vi "FTW-Test.vi"() -> ()   [LabVIEW 2014]
uses:
  src/core/time/FTW-Time-DisplayFormat-Timestamp.ctl
  src/core/error/FTW-ERR-ExceptionType.ctl
  src/core/time/FTW-Time-Uptime.vi
  src/core/reflection/FTW-Reflection-Type.vi
  lib/jansson/FTWLib-JSON-LibraryFilepath.vi
  src/core/json/lib/FTW-JSON-Core-LibraryError.vi
  src/core/json/lib/FTW-JSON-Core-ElementType.vi
  src/core/error/FTW-ERR-ThrowGenericError.vi
  src/core/json/lib/FTW-JSON-Core-EncodingFlags.vi
  src/core/error/FTW-ERR-ThrowError.vi
  src/core/error/FTW-ERR-CallChain.vi
  src/core/string/FTW-STR-ReplaceWhitespace.vi
  src/core/json/lib/FTW-JSON-Core-GetFlattenedValue.vi
  src/core/sync/barrier/FTW-Sync-Synchronizer.xnode
  src/core/json/FTW-JSON-Deserialize/FTW-JSON-Deserialize.xnode
  src/core/array/shuffle/FTW-Array-Shuffle.xnode
  <vilib>/regexp/Match Regular Expression.xnode
  kernel32.dll
panel:
  out "Results":string
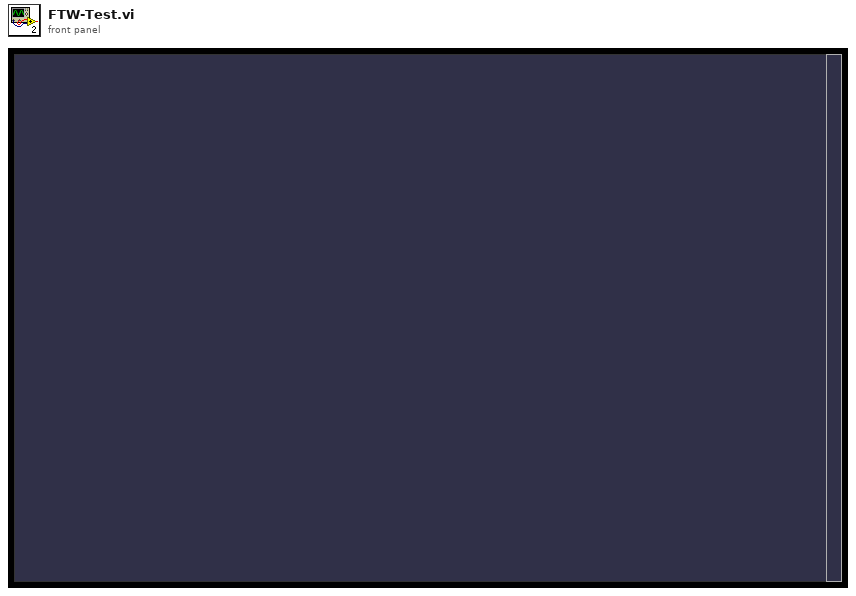
[diagram p1: front panel]
types:
  T1 = typedef "FTW-Time-DisplayFormat-Timestamp.ctl" = enum16{"YYYY-MM-DDT00:00:00.000Z (ISO-8601)", "YYYY-MM-DDT00-00-00Z (Simple ISO-8601)", "YYYY-MM-DD"}
  T2 = cluster{"Randomize Test Order":bool, "Tests Directory":path, "Test Configuration":cluster{"Default":cluster{"Enable":bool, "Iterations":i32}}, "Test Configuration":string, "Test Worker Pool Size":i32}
  T3 = enum32{"invalid app kind", "Development System", "Run Time System", "Student Edition", "Embedded LabVIEW", "Evaluation", "Custom"}
  T4 = enum32{"invalid CPU target", "Motorola 68K", "PowerPC", "Intel x86", "SPARC", "PA-RISC", "MIPS", "Alpha", "ARM", "AMD/Intel x64"}
  T5 = typedef "FTW-ERR-ExceptionType.ctl" = enum16{"OK", "Info", "Warning", "Error"}
  T6 = cluster{"Execute?":bool, "TestName":string, "MinTime":dbl, "MeanTime":dbl, "MaxTime":dbl, "Runs":i32, "Result":T5, "Hint":string, "TotalTime":dbl}
  T7 = enum32{"Bad", "Idle", "Run top level", "Running"}
  T8 = cluster{"VIRef":refnum<vi>, "TestName":string, "TestInstance":i32, "TestPoolSize":i32, "TestID":i32}
  T9 = cluster{"Color":u32, "Text":string, "Comment":string}[]
  T10 = cluster{"Color":u32, "Text":string, "Comment":string}
  T11 = cluster{u32, "offset past match":u32, "Color":u32}[]
  T12 = cluster{"VIRef":refnum<vi>, "TestName":string, "TestInstance":i32, "TestPoolSize":i32, "TestID":i32}[]
  T13 = cluster{"TestID":i32, "ElapsedTime":dbl, "Result":T5}
  T14 = cluster{"Execute?":bool, "TestName":string, "MinTime":dbl, "MeanTime":dbl, "MaxTime":dbl, "Runs":i32, "Result":T5, "Hint":string, "TotalTime":dbl}[]
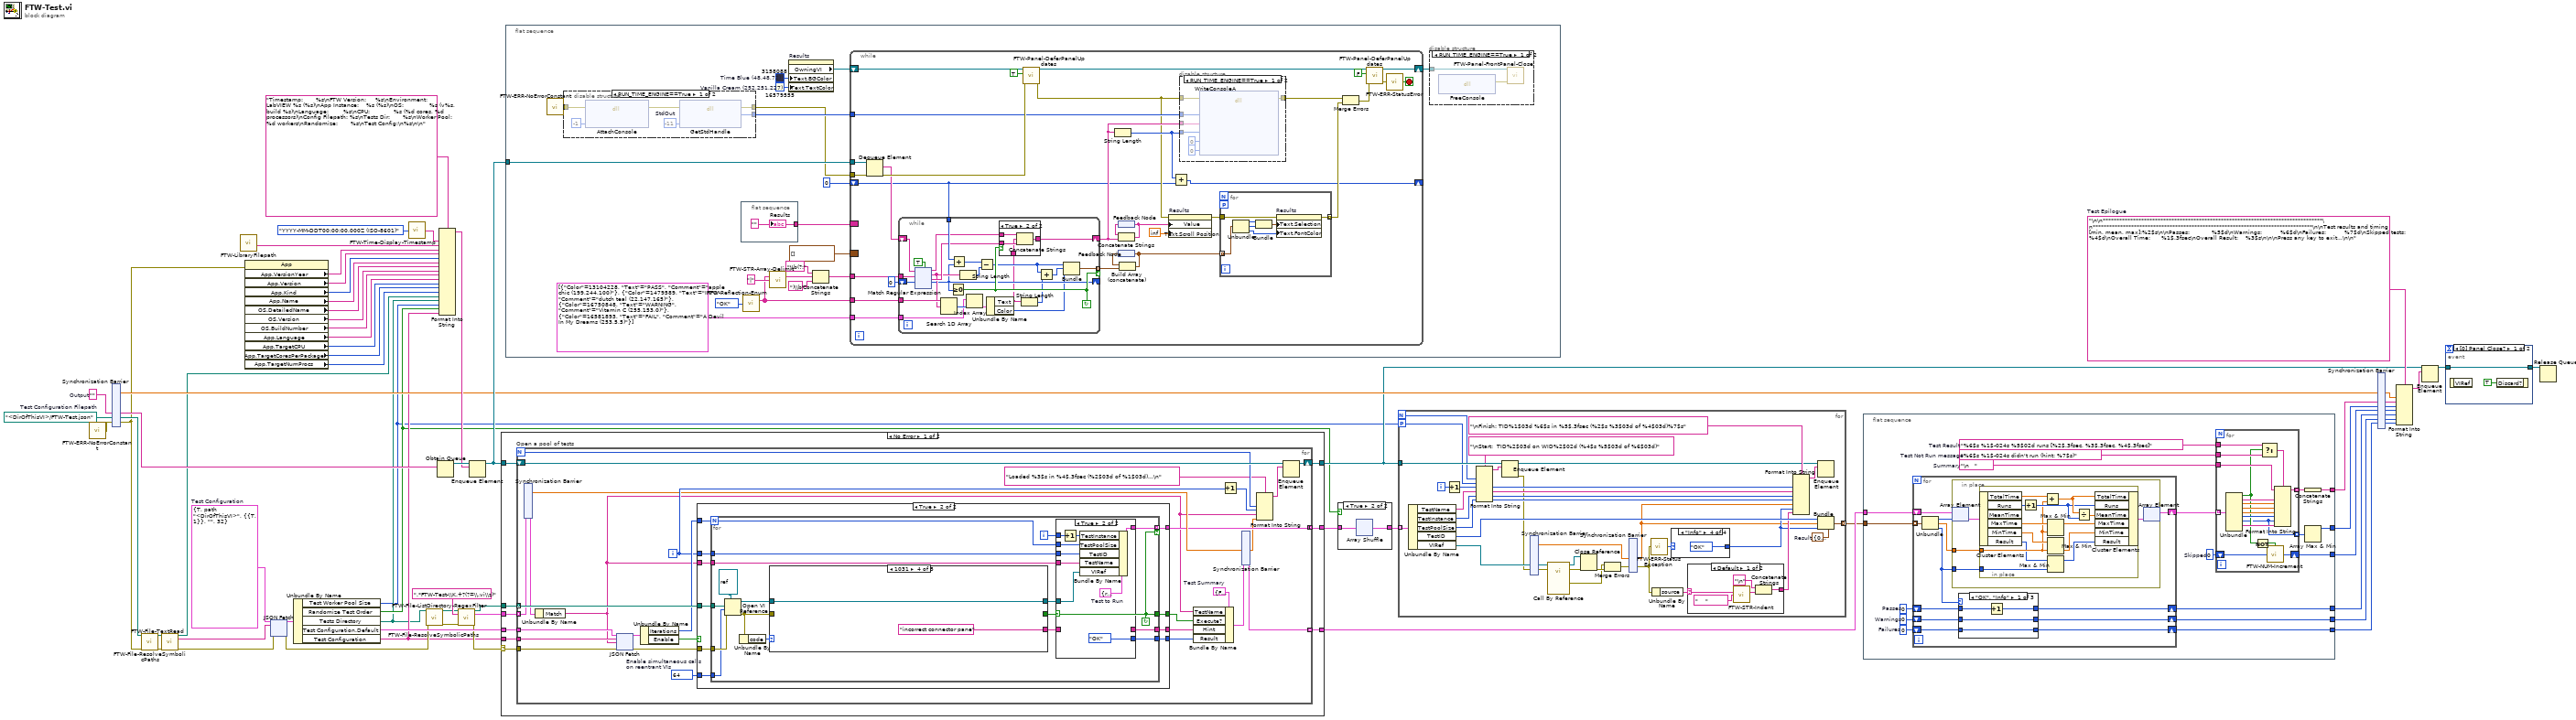
[diagram p0: block diagram]
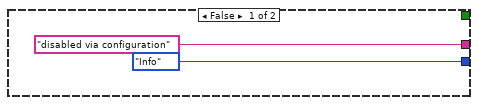
[diagram p5: hidden frame]
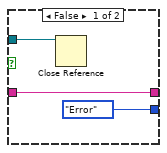
[diagram p6: hidden frame]
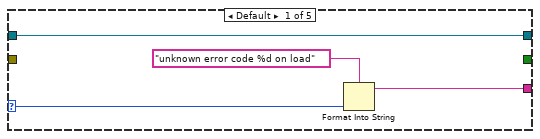
[diagram p7: hidden frame]
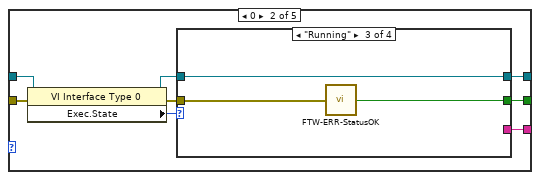
[diagram p8: hidden frame]
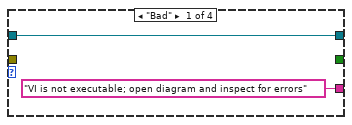
[diagram p9: hidden frame]
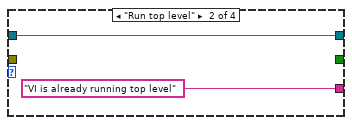
[diagram p10: hidden frame]
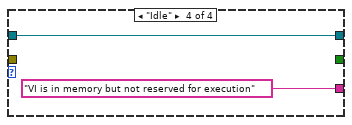
[diagram p11: hidden frame]
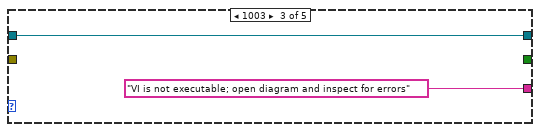
[diagram p12: hidden frame]
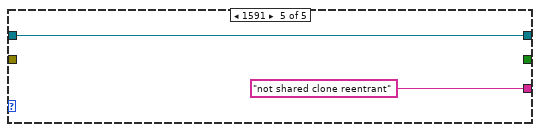
[diagram p13: hidden frame]
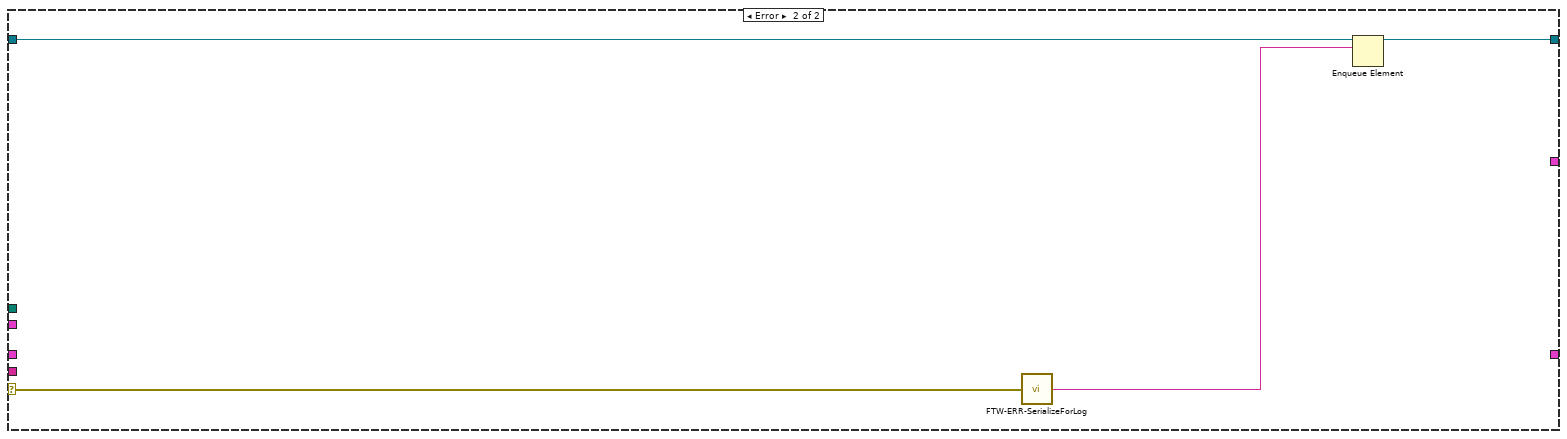
[diagram p14: hidden frame]
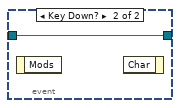
[diagram p19: hidden frame]
diagram:
  w55 = "\n\n********************************************************************************\n********************************************************************************\n\nTest results and timing [min, mean, max]:%2$s\n\nPasses:            %5$d\nWarnings:          %6$d\nFailures:          %7$d\nSkipped tests:     %4$d\nOverall Time:      %1$.3fsec\nOverall Result:    %3$s\n\n\nPress any key to exit...\n\n"  # Test Epilogue
  w38 = path "<DirOfThisVI>/FTW-Test.json"  # Test Configuration Filepath
  w35 = T2 {"Randomize Test Order"=TRUE, "Tests Directory"=path "<DirOfThisVI>", "Test Configuration"={"Default"={"Enable"=TRUE, "Iterations"=1}}, "Test Configuration"="", "Test Worker Pool Size"=32}  # Test Configuration
  w39 = ""  # Output
  n1 = call "FTW-ERR-NoErrorConstant.vi"() -> ("no error"=w11:errorcluster)
  n2 = xnode "Synchronization Barrier"("Synchronized Signal 1"=w39, "Synchronized Signal 2"=w38, "Synchronized Signal 3"=w11) -> ("High-Resolution Timer"=w16:dbl, w36:string, w37:path, w10:errorcluster)  [unwired: 1 in, 1 out]
  n3 = call "FTW-File-ResolveSymbolicPaths.vi"("Unresolved Path"=w37, "error in"=w10) -> ("Resolved Path"=w18:path, "error out"=w56:errorcluster)  [unwired: 12 in]
  n4 = call "FTW-File-TextRead.vi"("Filepath"=w18, "error in"=w56) -> ("Filepath out"=w8:path, "Text"=w31:string, "error out"=w33:errorcluster)  [unwired: 11 in]
  n5 = call "FTW-LibraryFilepath.vi"() -> ("Library Version"=w6:string)  [unwired: 9 in, 2 out]
  n6 = property class="App"(error in=w10) -> ("App.VersionYear"=w30:string, "App.Version"=w28:string, "App.Kind"=w20:T3, "App.Name"=w19:string, "OS.DetailedName"=w29:string, "OS.Version"=w27:string, "OS.BuildNumber"=w26:string, "App.Language"=w25:string, "App.TargetCPU"=w24:T4, "App.TargetCoresPerPackage"=w23:i32, "App.TargetNumProcs"=w21:i32)  [unwired: 1 in, 2 out]
  n7 = xnode "JSON Fetch"("Type and Defaults"=w35, "JSON String"=w31, "error in"=w33) -> ("Values"=w34:T2, "error out"=w32:errorcluster)  [unwired: 1 in]
  n8 = Unbundle By Name(w34) -> ("Test Worker Pool Size"=w3:i32, "Randomize Test Order"=w7:bool, "Tests Directory"=w4:path, "Test Configuration.Default"=w61:cluster{"Enable":bool, "Iterations":i32}, "Test Configuration"=w9:string)
  n9 = call "FTW-Time-Display-Timestamp.vi"("Format"=FTW-Time-DisplayFormat-Timestamp."YYYY-MM-DDT00:00:00.000Z (ISO-8601)") -> ("Formatted Timestamp"=w15:string)  [unwired: 3 in]
  n10 = call "FTW-File-ResolveSymbolicPaths.vi"("Unresolved Path"=w4, "error in"=w32) -> ("Resolved Path"=w5:path, "error out"=w62:errorcluster)  [unwired: 12 in]
  n11 = Obtain Queue(element data type=w36) -> (queue out=w57:refnum<queue>)  [unwired: 4 in, 2 out]
  n12 = Format Into String(format string="Timestamp:       %s\nFTW Version:     %s\nEnvironment:     LabVIEW %s (%s)\nApp Instance:    %s (%s)\nOS:              %s (v%s, build %s)\nLanguage:        %s\nCPU:             %s (%d cores, %d processors)\nConfig Filepath: %s\nTests Dir:       %s\nWorker Pool:     %d workers\nRandomize:       %s\nTest Config:\n%s\n\n", w15, w6, w30, w28, w20, w19, w29, w27, w26, w25, w24, w23, w21, w8, w4, w3, w7, w9) -> (resulting string=w17:string)  [unwired: 2 in, 1 out]
  n13 = call "FTW-File-ListDirectory-RegexFilter.vi"("Directory to Search"=w5, "Filename Regex Filter"=".*FTW-Test-\\K.+?(?=\\.vi\\z)", "error in"=w62) -> ("Matching Filepaths"=w64:path[], "Regex Results"=w65:cluster{"Match":string, "Submatches":string[]}[], "error out"=w54:errorcluster)  [unwired: 9 in, 1 out]
  n14 = Enqueue Element(queue=w57, element=w17) -> (queue out=w53:refnum<queue>)  [unwired: 2 in, 2 out]
  n15 = case shown="No Error" w54 {
    selector: w54 -> [w71 w253]
    tunnel: w65 -> [w75 _]
    tunnel: w64 -> [w74 _]
    tunnel: [w67 _] -> w12
    tunnel: w61 -> [w73 _]
    tunnel: w9 -> [w72 _]
    tunnel: [w70 _] -> w60
    tunnel: w53 -> [w69 w250]
    tunnel: [w68 w252] -> w13
    frame No Error {
      n16 = for "Open a pool of tests" {
        N -> [w97]
        tunnel: w71 -> [w93]
        tunnel: [w87] -> w67 mode=concatenating
        tunnel: w75 -> [w90] mode=indexing
        tunnel: w74 -> [w103] mode=indexing
        tunnel: [w85] -> w70 mode=indexing
        tunnel: w73 -> [w95]
        tunnel: w72 -> [w94]
        shift-right: [w83] -> w68
        shift-left: w69 -> [w99]
        i -> [w96]
        w81 = 64  # Enable simultaneous calls on reentrant VIs
        w100 = T6 {"Execute?"=FALSE, "TestName"="", "MinTime"=inf, "MeanTime"=0.0, "MaxTime"=-inf, "Runs"=0, "Result"=enum."OK", "Hint"="", "TotalTime"=0.0}  # Test Summary
        n17 = xnode "Synchronization Barrier"("Synchronized Signal 1"=w90) -> ("High-Resolution Timer"=w88:dbl, w89:cluster{"Match":string, "Submatches":string[]})  [unwired: 1 in, 1 out]
        n18 = Unbundle By Name(w89) -> ("Match"=w78:string)
        n19 = xnode "JSON Fetch"("Type and Defaults"=w95, "JSON String"=w94, "Element Path"=w78, "error in"=w93) -> ("Values"=w91:cluster{"Enable":bool, "Iterations":i32}, "error out"=w92:errorcluster)
        n20 = Unbundle By Name(w91) -> ("Iterations"=w101:i32, "Enable"=w77:bool)
        n21 = case shown="True" w77 {
          tunnel: w103 -> [_ w193]
          tunnel: w81 -> [_ w192]
          tunnel: [_ w191] -> w87
          tunnel: w96 -> [_ w190]
          tunnel: ["disabled via configuration" w189] -> w102
          tunnel: w101 -> [_ w188]
          tunnel: w92 -> [_ w187]
          tunnel: w78 -> [_ w186]
          tunnel: [FTW-ERR-ExceptionType."Info" ("Result") w185] -> w82
          tunnel: [_ w184] -> w76
          frame False {
          }
          frame True {
            n22 = for {
              N: w188 -> [w202]
              tunnel: w187 -> [w210]
              tunnel: w193 -> [w209]
              tunnel: w192 -> [w208]
              tunnel: w186 -> [w204]
              tunnel: [w201] -> w191 mode=indexing if=w194
              tunnel: [w197] -> w189
              tunnel: w190 -> [w196]
              tunnel: [w195] -> w185
              tunnel: [w194] -> w184
              i -> [w203]
              stop <- w194 continue-if-true
              n23 = Open VI Reference(type specifier VI Refnum (for type only)=refnum<vi> refnum, vi path=w209, options=w208, error in (no error)=w210) -> (vi reference=w200:refnum<vi>, error out=w206:errorcluster)  [unwired: 2 in]
              n24 = Unbundle By Name(w206) -> ("code"=w205:i32)
              n25 = case shown="1031" w205 {
                selector: w205 -> [w225 _ _ _ _]
                tunnel: w200 -> [w223 w234 w244 w246 w248]
                tunnel: w206 -> [_ w233 _ _ _]
                tunnel: [_ w230 _ _ _] -> w194
                tunnel: [w224 w228 "VI is not executable; open diagram and inspect for errors" "incorrect connector pane" "not shared clone reentrant"] -> w198
                tunnel: [w223 w227 w244 w246 w248] -> w199
                frame Default {
                  n26 = Format Into String(format string="unknown error code %d on load", w225) -> (resulting string=w224:string)  [unwired: 2 in, 1 out]
                }
                frame 0 {
                  n27 = property class="VI Interface Type 0"(reference=w234, error in=w233) -> (reference out=w231:refnum<vi>, error out=w232:errorcluster, "Exec.State"=w229:T7)
                  n28 = case shown="\"Running\"" w229 {
                    tunnel: w232 -> [_ _ w240 _]
                    tunnel: w231 -> [w235 w237 w241 w243]
                    tunnel: [_ _ w239 _] -> w230
                    tunnel: ["VI is not executable; open diagram and inspect for errors" "VI is already running top level" _ "VI is in memory but not reserved for execution"] -> w228
                    tunnel: [w235 w237 w241 w243] -> w227
                    frame "Bad" {
                    }
                    frame "Run top level" {
                    }
                    frame "Running" {
                      n29 = call "FTW-ERR-StatusOK.vi"("error to check"=w240) -> ("Status OK?"=w239:bool)
                    }
                    frame "Idle" {
                    }
                  }
                }
                frame 1003 {
                }
                frame 1031 {
                }
                frame 1591 {
                }
              }
              n30 = case shown="True" w194 {
                tunnel: w199 -> [w213 w222]
                tunnel: w204 -> [_ w216]
                tunnel: w203 -> [_ w221]
                tunnel: w202 -> [_ w219]
                tunnel: [_ w220] -> w201
                tunnel: w198 -> [w212 _]
                tunnel: [w212 _] -> w197
                tunnel: w196 -> [_ w218]
                tunnel: [FTW-ERR-ExceptionType."Error" ("Result") FTW-ERR-ExceptionType."OK" ("Result")] -> w195
                frame False {
                  n31 = Close Reference(reference=w213) -> ()  [unwired: 1 in, 1 out]
                }
                frame True {
                  w217 = T8 {"VIRef"=refnum, "TestName"="", "TestInstance"=0, "TestPoolSize"=0, "TestID"=0}  # Test to Run
                  n32 = Increment(x=w221) -> (x+1=w215:i32)
                  n33 = Bundle By Name(cluster=w217, "TestInstance"=w215, "TestPoolSize"=w219, "TestID"=w218, "TestName"=w216, "VIRef"=w222) -> (w220:T8)
                }
              }
            }
          }
        }
        n34 = Bundle By Name(cluster=w100, "TestName"=w78, "Execute?"=w76, "Hint"=w102, "Result"=w82) -> (w86:T6)
        n35 = Increment(x=w96) -> (x+1=w79:i32)
        n36 = xnode "Synchronization Barrier"("Upstream Timer Value"=w88, "Synchronized Signal 1"=w86) -> ("Elapsed Time"=w84:dbl, w85:T6)  [unwired: 1 out]
        n37 = Format Into String(format string="Loaded %3$s in %4$.3fsec (%2$03d of %1$03d)...\n", w97, w79, w78, w84) -> (resulting string=w98:string)  [unwired: 2 in, 1 out]
        n38 = Enqueue Element(queue=w99, element=w98) -> (queue out=w83:refnum<queue>)  [unwired: 2 in, 2 out]
      }
    }
    frame Error {
      n39 = call "FTW-ERR-SerializeForLog.vi"("error in"=w253) -> ("Serialized Error"=w251:string)
      n40 = Enqueue Element(queue=w250, element=w251) -> (queue out=w252:refnum<queue>)  [unwired: 2 in, 2 out]
    }
  }
  n41 = flat-sequence {
    tunnel: w53 -> [w272]
    frame #0 {
      w268 = u32 16579555  # Vanilla Cream (252,251,227)
      w269 = u32 3158088  # Time Blue (48,48,72)
      n42 = call "FTW-ERR-NoErrorConstant.vi"() -> ("no error"=w257:errorcluster)
      n43 = disable-structure shown="RUN_TIME_ENGINE==True" {
        disable-tunnel: w257 -> [w278 w282]
        disable-tunnel: [w277 w282] -> w254
        disable-tunnel: [w276 _] -> w260
        frame condition #0 {
          w280 = -11  # StdOut
          n44 = dll-call lib="kernel32.dll" fn="AttachConsole"(error in=w278, "arg1"=-1) -> (error out=w281:errorcluster)  [unwired: 4 in, 1 out]
          n45 = dll-call lib="kernel32.dll" fn="GetStdHandle"(error in=w281, "nStdHandle"=w280) -> (error out=w277:errorcluster, "return type"=w276:i32)  [unwired: 3 in, 1 out]
        }
        frame condition #1 (active) {
        }
      }
      n46 = flat-sequence {
        tunnel: [w275] -> w258
        frame #0 {
          w275 = "" ("Results")
          "Results" <- w275
        }
      }
      n47 = call "FTW-Reflection-Enum.vi"("Enum"=FTW-ERR-ExceptionType."OK" ("Exception")) -> ("Enum Items"=w262:string[])  [unwired: 12 in, 2 out]
      n48 = call "FTW-STR-Array-Delimit.vi"("Array of Strings"=w262, "Delimiter"="|") -> ("Delimited String"=w264:string)  [unwired: 13 in]
      n49 = property on="Results" class="Str"("Text.BGColor"=w269, "Text.TextColor"=w268) -> ("OwningVI"=w267:refnum<vi>)  [unwired: 2 in, 2 out]
      n50 = Concatenate Strings("\\b(?:" ("string"), w264, ")\\b" ("string")) -> (w263:string)
      n51 = while {
        tunnel: w260 -> [w300]
        tunnel: w263 -> [w311]
        border: cluster{u32, "offset past match":u32, u32}[] [] -> [_]
        border: w258 -> [_]
        tunnel: w262 -> [w310]
        tunnel: T9 [{"Color"=13104228, "Text"="PASS", "Comment"="apple chic (199,244,100)"}, {"Color"=1479589, "Text"="INFO", "Comment"="dutch teal (22,147,165)"}, {"Color"=16750848, "Text"="WARNING", "Comment"="Vitamin C (255,153,0)"}, {"Color"=16581893, "Text"="FAIL", "Comment"="A Devil In My Dreams (253,5,5)"}] -> [w298]
        shift-right: [w297] -> w259
        shift-left: w267 -> [w309]
        tunnel: w272 -> [w313]
        tunnel: w254 -> [w293]
        shift-right: [w284] -> _
        shift-left: 0 ("length") -> [w285]
        stop <- w296 stop-if-true
        n52 = Dequeue Element(queue=w313, error in (no error)=w293) -> (element=w295:string, error out=w312:errorcluster)  [unwired: 1 in, 2 out]
        n53 = while {
          shift-right: [w336] -> _
          shift-left: 0 ("offset past match") -> [w350]
          tunnel: w311 -> [w351]
          tunnel: [w345] -> w306 mode=indexing if=w340
          tunnel: w285 -> [w348]
          tunnel: w310 -> [w347]
          shift-right: [w342] -> w299
          shift-left: w295 -> [w344]
          tunnel: w298 -> [w338]
          stop <- w340 continue-if-true
          n54 = xnode "Match Regular Expression"("input string"=w344, "regular expression"=w351, "offset (0)"=w350, "multiline? (F)"=TRUE) -> ("before match"=w343:string, "whole match"=w337:string, "after match"=w341:string, "offset past match"=w336:i32)  [unwired: 2 in, 1 out]
          n55 = Search 1D Array(1D array=w347, element=w337) -> (index of element=w339:i32)  [unwired: 1 in]
          n56 = Greater Or Equal To 0?(x=w336) -> (x >= 0?=w340:bool)
          n57 = Add(x=w348, y=w336) -> (x+y=w346:i32)
          n58 = String Length(string=w337) -> (length=w335:i32)
          n59 = Index Array(array=w338, index=w339) -> (element=w331:T10)
          n60 = Subtract(x=w346, y=w335) -> (x-y=w334:i32)
          n61 = Unbundle By Name(w331) -> ("Text"=w330:string, "Color"=w329:u32)
          n62 = case shown="True" w340 {
            tunnel: w343 -> [w352 w356]
            tunnel: [w352 w355] -> w342
            tunnel: w341 -> [_ w354]
            tunnel: w330 -> [_ w353]
            frame False {
            }
            frame True {
              n63 = Concatenate Strings(w356, w353, w354) -> (w355:string)
            }
          }
          n64 = String Length(string=w330) -> (length=w332:i32)
          n65 = Add(x=w334, y=w332) -> (x+y=w333:i32)
          n66 = Bundle(w334, w333, "Color"=w329) -> (w345:cluster{i32, i32, "Color":u32})  [unwired: 1 in]
        }
        n67 = call "FTW-Panel-DeferPanelUpdates.vi"("error in"=w312, "Defer?"=TRUE, "VI Ref"=w309) -> ("error out"=w290:errorcluster, "VI Ref out"=w302:refnum<vi>)  [unwired: 7 in]
        n68 = String Length(string=w299) -> (length=w292:i32)
        n69 = feedback #1() -> (w304:string)
        n70 = Concatenate Strings(w304, w299) -> (w305:string)
        n71 = feedback-in #1(w305) -> ()
        n72 = feedback #2() -> (w307:cluster{u32, "offset past match":u32, u32}[])
        n73 = Build Array (concatenate)(w307, w306) -> (w291:T11)
        n74 = feedback-in #2(w291) -> ()
        n75 = property on="Results" class="Str"(error in=w290, "Value"=w305, "Text.Scroll Position"=inf) -> (error out=w289:errorcluster)  [unwired: 1 in, 1 out]
        n76 = Add(x=w292, y=w285) -> (x+y=w284:i32)
        n77 = disable-structure shown="RUN_TIME_ENGINE==True" {
          disable-tunnel: w300 -> [w318 _]
          disable-tunnel: [w317 w321] -> w286
          disable-tunnel: w290 -> [w316 w321]
          disable-tunnel: w299 -> [w315 _]
          disable-tunnel: w292 -> [w314 _]
          frame condition #0 {
            n78 = dll-call lib="kernel32.dll" fn="WriteConsoleA"(error in=w316, "hConsoleOutput"=w318, "lpBuffer"=w315, "numberOfCharsToWrite"=w314, "lpNumberOfCharsWritten"=0, "lpReserved"=0 ("lpNumberOfCharsWritten")) -> (error out=w317:errorcluster)  [unwired: 5 in, 4 out]
          }
          frame condition #1 (active) {
          }
        }
        n79 = for {
          tunnel: w291 -> [w328] mode=indexing
          workers-P: _ -> [_]
          tunnel: w289 -> [w323]
          tunnel: [w322] -> w288 mode=indexing
          n80 = Unbundle(w328) -> (w326:u32, "offset past match"=w325:u32, "Color"=w327:u32)
          n81 = Bundle(w326, "offset past match"=w325) -> (w324:cluster{u32, "offset past match":u32})  [unwired: 1 in]
          n82 = property on="Results" class="Str"(error in=w323, "Text.Selection"=w324, "Text.FontColor"=w327) -> (error out=w322:errorcluster)  [unwired: 1 in, 1 out]
        }
        n83 = Merge Errors(w286, w288) -> (w287:errorcluster)
        n84 = call "FTW-Panel-DeferPanelUpdates.vi"("error in"=w287, "Defer?"=FALSE, "VI Ref"=w302) -> ("error out"=w294:errorcluster, "VI Ref out"=w297:refnum<vi>)  [unwired: 7 in]
        n85 = call "FTW-ERR-StatusError.vi"("error to check"=w294) -> ("Error?"=w296:bool)
      }
      n86 = disable-structure shown="RUN_TIME_ENGINE==True" {
        disable-tunnel: w259 -> [w273 _]
        frame condition #0 {
          n87 = dll-call lib="kernel32.dll" fn="FreeConsole"() -> (error out=w274:errorcluster)  [unwired: 3 in, 2 out]
          n88 = call "FTW-Panel-FrontPanel-Close.vi"("error in"=w274, "VI Ref"=w273) -> ()  [unwired: 8 in, 2 out]
        }
        frame condition #1 (active) {
        }
      }
    }
  }
  n89 = case shown="True" w7 {
    tunnel: [w471 w472] -> w1
    tunnel: w12 -> [w471 w473]
    frame False {
    }
    frame True {
      n90 = xnode "Array Shuffle"("Array"=w473) -> ("Shuffled Array"=w472:T12)
    }
  }
  n91 = for {
    N -> [w504]
    tunnel: w1 -> [w522] mode=indexing
    workers-P: w3 -> [w505]
    tunnel: [w514] -> w2 mode=indexing
    tunnel: w13 -> [w521]
    i -> [w519]
    w499 = T13 {"TestID"=0, "ElapsedTime"=0.0, "Result"=enum."OK"}  # Result
    n92 = Unbundle By Name(w522) -> ("TestName"=w518:string, "TestInstance"=w517:i32, "TestPoolSize"=w516:i32, "TestID"=w515:i32, "VIRef"=w498:refnum<vi>)
    n93 = Increment(x=w519) -> (x+1=w503:i32)
    n94 = Format Into String(format string="\nStart:  TID%2$03d on WID%2$02d (%4$s %5$03d of %6$03d)", w504, w505, w503, w518, w517, w516) -> (resulting string=w520:string)  [unwired: 2 in, 1 out]
    n95 = Enqueue Element(queue=w521, element=w520) -> (queue out=w500:refnum<queue>, error out=w497:errorcluster)  [unwired: 2 in, 1 out]
    n96 = xnode "Synchronization Barrier"("Synchronized Signal 1"=w498, "Synchronized Signal 2"=w497) -> ("High-Resolution Timer"=w494:dbl, w496:refnum<vi>, w495:errorcluster)  [unwired: 1 in, 1 out]
    n97 = call-by-ref "?"(reference=w496, error in=w495) -> (reference out=w513:refnum<vi>, error out=w512:errorcluster, "Test Result"=w510:errorcluster)
    n98 = Close Reference(reference=w513, error in (no error)=w512) -> (error out=w511:errorcluster)
    n99 = Merge Errors(w510, w511) -> (w493:errorcluster)
    n100 = xnode "Synchronization Barrier"("Upstream Timer Value"=w494, "Synchronized Signal 1"=w493) -> ("Elapsed Time"=w491:dbl, w492:errorcluster)  [unwired: 1 out]
    n101 = call "FTW-ERR-StatusException.vi"("error to check"=w492) -> ("Exception"=w502:T5)
    n102 = Unbundle By Name(w492) -> ("source"=w509:string)
    n103 = case shown="\"Info\"" w502 {
      selector: w502 -> [w533 w534 w535 _]
      tunnel: [w533 w534 w535 FTW-ERR-ExceptionType."OK" ("Result")] -> w501
      frame "OK" {
      }
      frame "Warning" {
      }
      frame "Error" {
      }
      frame "Info" {
      }
    }
    n104 = case shown="Default" w509 {
      selector: w509 -> [w539 w542]
      tunnel: [w540 w542] -> w508
      frame Default {
        n105 = call "FTW-STR-Indent.vi"("String"=w539, "Indentation Characters"="    ") -> ("Indented String"=w538:string)  [unwired: 13 in]
        n106 = Concatenate Strings("\n", w538) -> (w540:string)
      }
      frame "" {
      }
    }
    n107 = Format Into String(format string="\nFinish: TID%1$03d %6$s in %5$.3fsec (%2$s %3$03d of %4$03d)%7$s", w503, w518, w517, w516, w491, w501, w508) -> (resulting string=w523:string)  [unwired: 2 in, 1 out]
    n108 = Bundle(cluster=w499, "TestID"=w515, "ElapsedTime"=w491, "Result"=w501) -> (w514:T13)
    n109 = Enqueue Element(queue=w500, element=w523) -> ()  [unwired: 2 in, 3 out]
  }
  n110 = flat-sequence {
    tunnel: w2 -> [w560]
    tunnel: w60 -> [w559]
    tunnel: [w549] -> w51
    tunnel: [w548] -> w50
    tunnel: [w547] -> w47
    tunnel: [w546] -> w45
    tunnel: [w545] -> w44
    tunnel: [w544] -> w42
    frame #0 {
      w543 = "\n   "  # Summary
      w550 = 0  # Failures
      w551 = 0  # Warnings
      w552 = 0  # Passes
      w553 = "%6$s %1$-024s %5$02d runs [%2$.3fsec, %3$.3fsec, %4$.3fsec]"  # Test Result
      w554 = "%6$s %1$-024s didn't run (hint: %7$s)"  # Test Not Run message
      w555 = 0  # Skipped
      n111 = for {
        tunnel: w560 -> [w587] mode=indexing
        shift-right: [w588] -> w558
        shift-left: w559 -> [w589]
        shift-right: [w579] -> w549
        shift-left: w550 -> [w578]
        shift-right: [w581] -> w548
        shift-left: w551 -> [w580]
        shift-right: [w582] -> w547
        shift-left: w552 -> [w583]
        n112 = Unbundle(w587) -> ("TestID"=w586:i32, "ElapsedTime"=w585:dbl, "Result"=w584:T5)
        n113 = in-place {
          in-place-border: w585 -> [w601]
          in-place-border: w584 -> [w600]
          n114 = in-place-array #3(w589, w586) -> (w603:T6)
          n115 = in-place {
            in-place-border: w601 -> [w608]
            in-place-border: w600 -> [w604]
            n116 = in-place-cluster #4(w603) -> ("TotalTime"=w616:dbl, "Runs"=w615:i32, "MaxTime"=w611:dbl, "MinTime"=w609:dbl, "Result"=w606:T5)  [unwired: 1 out]
            n117 = Increment(x=w615) -> (x+1=w613:i32)
            n118 = Add(x=w616, y=w608) -> (x+y=w614:dbl)
            n119 = Max & Min(x=w611, y=w608) -> (max(x,y)=w610:dbl)  [unwired: 1 out]
            n120 = Max & Min(x=w609, y=w608) -> (min(x,y)=w607:dbl)  [unwired: 1 out]
            n121 = Max & Min(x=w606, y=w604) -> (max(x,y)=w605:u16)  [unwired: 1 out]
            n122 = Divide(x=w614, y=w613) -> (x/y=w612:dbl)
            n123 = in-place-cluster #4("TotalTime"=w614, "Runs"=w613, "MeanTime"=w612, "MaxTime"=w610, "MinTime"=w607, "Result"=w605) -> (w602:T6)
          }
          n124 = in-place-array #3(w602) -> (w588:T14)  [unwired: 1 out]
        }
        n125 = case shown="\"OK\", \"Info\"" w584 {
          tunnel: w583 -> [w593 w596 w599]
          tunnel: [w590 w596 w599] -> w582
          tunnel: [w592 w595 w598] -> w581
          tunnel: w580 -> [w592 w595 w598]
          tunnel: [w591 w594 w597] -> w579
          tunnel: w578 -> [w591 w594 w597]
          frame "OK", "Info" {
            n126 = Increment(x=w593) -> (x+1=w590:i32)
          }
          frame "Warning" {
          }
          frame "Error" {
          }
        }
      }
      n127 = for {
        tunnel: w558 -> [w565] mode=indexing
        tunnel: [w577] -> w557 mode=indexing
        tunnel: w553 -> [w572]
        tunnel: w554 -> [w571]
        tunnel: [w561] -> w556 mode=indexing
        shift-right: [w567] -> w546
        shift-left: w555 -> [w568]
        tunnel: w543 -> [w566]
        n128 = Unbundle(w565) -> ("Execute?"=w563:bool, "TestName"=w576:string, "MinTime"=w575:dbl, "MeanTime"=w574:dbl, "MaxTime"=w573:dbl, "Runs"=w569:i32, "Result"=w561:T5, "Hint"=w564:string)  [unwired: 1 out]
        n129 = Not(x=w563) -> (.not. x?=w562:bool)
        n130 = Select(t=w572, s=w563, f=w571) -> (s? t:f=w570:string)
        n131 = call "FTW-NUM-Increment.vi"("Initial Value"=w568, "Increment?"=w562) -> ("Final Value"=w567:i32)
        n132 = Format Into String(format string=w570, initial string=w566, w576, w575, w574, w573, w569, w561, w564) -> (resulting string=w577:string)  [unwired: 1 in, 1 out]
      }
      n133 = Concatenate Strings(w557) -> (w544:string)
      n134 = Array Max & Min(array=w556) -> (max value=w545:T5)  [unwired: 3 out]
    }
  }
  n135 = xnode "Synchronization Barrier"("Upstream Timer Value"=w16, "Synchronized Signal 1"=w42, "Synchronized Signal 1"=w44, "Synchronized Signal 2"=w45, "Synchronized Signal 3"=w47, "Synchronized Signal 4"=w50, "Synchronized Signal 5"=w51) -> ("Elapsed Time"=w52:dbl, w41:string, w43:T5, w40:i32, w46:i32, w48:i32, w49:i32)  [unwired: 1 out]
  n136 = Format Into String(format string=w55, w52, w41, w43, w40, w46, w48, w49) -> (resulting string=w63:string)  [unwired: 2 in, 1 out]
  n137 = Enqueue Element(queue=w13, element=w63) -> (queue out=w59:refnum<queue>)  [unwired: 2 in, 2 out]
  n138 = event shown="[0] Panel Close?" {
    selector: _ -> [_ _]
    dyn-events: _ -> [_ _]
    timeout: _ -> [_ _]
    tunnel: w59 -> [w617 w619]
    tunnel: [w617 w619] -> w58
    event Panel Close? {
      n139 = event-data() -> ()  [unwired: 1 in, 1 out]
      n140 = event-data("Discard?"=TRUE) -> ()  [unwired: 1 in, 1 out]
    }
    event Key Down? {
      n141 = event-data() -> ()  [unwired: 1 in, 1 out]
      n142 = event-data() -> ()  [unwired: 2 in, 1 out]
    }
  }
  n143 = Release Queue(queue=w58) -> ()  [unwired: 2 in, 3 out]
